vi "HFRR ADV v04.vi"() -> ()   [LabVIEW 2025] (continued)
            n1293 = Compound Arithmetic op=OR(w1606, w1605) -> (w1604:bool)
            n1294 = Not A Number/Path/Refnum?(number/path/refnum=w1590) -> (NaN/Path/Refnum?=w1601:bool)
            n1295 = case shown="True" w1604 {
              frame False {
              }
              frame True {
                n1296 = local write "TEMP"(0.0 ("TEMP")) -> ()
                n1297 = local write "FF 2"(0.0 ("FF 2")) -> ()
                n1298 = local write "reinit"(TRUE ("reinit")) -> ()
              }
            }
            n1299 = Select(t=0.0, s=w1601, f=w1590) -> (s? t:f=w1589:dbl)
            "COF 2" <- w1589
            n1300 = local write "COF 3"(w1589) -> ()
          }
        }
      }
    }
    n1301 = Wait (ms)(milliseconds to wait=u32 50) -> ()  [unwired: 1 out]
    n1302 = local read "Quit"() -> (w1529:bool)
    "Rate" <- 2500.0 ("No of Samples")
  }
  n1303 = while {
    tunnel: w57 -> [_]
    tunnel: [w1641] -> _
    tunnel: [w1617] -> w56
    i -> [w1641]
    stop <- w1617 stop-if-true
    # "C:\\LAB-IQ-NXT\\Scar View.exe"
    n1304 = local read "OK Button 16"() -> (w1630:bool)
    n1305 = local read "Main Tab"() -> (w1623:T2)
    n1306 = local read "service 3"() -> (w1624:bool)
    n1307 = local read "OPEN 6"() -> (w1626:bool)
    n1308 = local read "EDIT 2"() -> (w1628:bool)
    n1309 = flat-sequence {
      frame #0 {
        n1310 = local read "SAVE 2"() -> (w2243:bool)
        n1311 = stacked-sequence {
          frame #0 {
            n1312 = local read "EDIT"() -> (w2297:bool)
            n1313 = case shown="True" w2297 {
              tunnel: [u8 2 ("Disabled") u8 0 ("Disabled")] -> _
              frame False {
                w2299 = FALSE
                n1314 = local write "Password"("") -> ()
                n1315 = property on="SrvM CP" class="Bool (strict)"("Visible"=w2299) -> ()  [unwired: 2 in, 2 out]
                n1316 = property on="message" class="Str"("Visible"=w2299) -> ()  [unwired: 2 in, 2 out]
                n1317 = local write "x = y?"(w2299) -> ()
                n1318 = property on="Password" class="Str"("Visible"=w2299) -> ()  [unwired: 2 in, 2 out]
                n1319 = property on="ENTER THE NEW PASSWORD" class="Str"("Visible"=w2299) -> ()  [unwired: 2 in, 2 out]
                n1320 = property on="ENTER CURRENT PASSWORD" class="Str"("Visible"=w2299) -> ()  [unwired: 2 in, 2 out]
                n1321 = local write "SrvM CP"(w2299) -> ()
              }
              frame True {
                w2302 = TRUE
                n1322 = property on="SrvM CP" class="Bool (strict)"("Visible"=w2302) -> ()  [unwired: 2 in, 2 out]
                n1323 = property on="Password" class="Str"("Visible"=w2302) -> ()  [unwired: 2 in, 2 out]
              }
            }
            "dipl pwd" <- "@143$\n" ("dipl pwd")
          }
          frame #1 {
            # "Gain password"
            n1324 = String To Byte Array(string="ENTER CURRENT PASSWORD") -> (unsigned byte array=w2307:u8[])
            n1325 = Search 1D Array(1D array=w2307, element=u8 10) -> (index of element=w2310:i32)  [unwired: 1 in]
            n1326 = Index Array(array=w2307, index=w2310) -> (element=w2306:u8)
            n1327 = Equal?(x=w2306, y=10) -> (x = y?=w2304:bool)
            n1328 = case shown="True" w2304 {
              frame False {
                n1329 = property on="ENTER THE NEW PASSWORD" class="Str"("Visible"=FALSE) -> ()  [unwired: 2 in, 2 out]
              }
              frame True {
                # "password"
                # "change password logic"
                n1330 = local read "ENTER CURRENT PASSWORD"() -> (w2323:string)
                n1331 = local read "dipl pwd"() -> (w2317:string)
                n1332 = String To Byte Array(string=w2323) -> (unsigned byte array=w2325:u8[])
                n1333 = String To Byte Array(string=w2317) -> (unsigned byte array=w2318:u8[])
                n1334 = Array Size(array=w2325) -> (size(s)=w2322:i32)
                n1335 = Array Size(array=w2318) -> (size(s)=w2320:i32)
                n1336 = for {
                  N: w2322 -> [_]
                  tunnel: w2325 -> [w2349]
                  tunnel: [w2347] -> w2326 mode=indexing
                  tunnel: w2322 -> [w2341]
                  i -> [w2342]
                  n1337 = Decrement(x=w2341) -> (x-1=w2339:i32)
                  n1338 = Equal?(x=w2342, y=w2339) -> (x = y?=w2340:bool)
                  n1339 = Index Array(array=w2349, index=w2342) -> (element=w2343:u8)
                  n1340 = Number To Decimal String(number=w2343) -> (decimal integer string=w2348:string)  [unwired: 1 in]
                  n1341 = Select(t="", s=w2340, f="\r") -> (s? t:f=w2345:string)
                  n1342 = Concatenate Strings(w2348, w2345) -> (w2347:string)
                }
                n1343 = for {
                  N: w2320 -> [_]
                  tunnel: w2318 -> [w2337]
                  tunnel: [w2335] -> w2319 mode=indexing
                  tunnel: w2320 -> [w2332]
                  i -> [w2333]
                  n1344 = Decrement(x=w2332) -> (x-1=w2331:i32)
                  n1345 = Equal?(x=w2333, y=w2331) -> (x = y?=w2330:bool)
                  n1346 = Index Array(array=w2337, index=w2333) -> (element=w2336:u8)
                  n1347 = Number To Decimal String(number=w2336) -> (decimal integer string=w2334:string)  [unwired: 1 in]
                  n1348 = Select(t="", s=w2330, f="\r") -> (s? t:f=w2327:string)
                  n1349 = Concatenate Strings(w2334, w2327) -> (w2335:string)
                }
                n1350 = local read "string"() -> (w2324:string)
                n1351 = Concatenate Strings(w2319) -> (w2313:string)
                n1352 = Concatenate Strings(w2324) -> (w2321:string)
                n1353 = Concatenate Strings(w2326) -> (w2314:string)
                n1354 = Equal?(x=w2314, y=w2321) -> (x = y?=w2316:bool)
                n1355 = Equal?(x=w2314, y=w2313) -> (x = y?=w2312:bool)
                n1356 = Or(x=w2316, y=w2312) -> (x .or. y?=w2315:bool)
                n1357 = case shown="True" w2315 {
                  frame False {
                  }
                  frame True {
                    n1358 = property on="ENTER THE NEW PASSWORD" class="Str"("Visible"=TRUE) -> ()  [unwired: 2 in, 2 out]
                  }
                }
              }
            }
          }
          frame #2 {
            n1359 = String To Byte Array(string="ENTER THE NEW PASSWORD") -> (unsigned byte array=w2352:u8[])
            n1360 = Search 1D Array(1D array=w2352, element=u8 10) -> (index of element=w2356:i32)  [unwired: 1 in]
            n1361 = Index Array(array=w2352, index=w2356) -> (element=w2354:u8)
            n1362 = Equal?(x=w2354, y=10) -> (x = y?=w2351:bool)
            n1363 = case shown="False" w2351 {
              frame False {
              }
              frame True {
                n1364 = local write "EDIT"(FALSE) -> ()
                n1365 = local write "SrvM CP"(FALSE) -> ()
                n1366 = local read "ENTER THE NEW PASSWORD"() -> (w2359:string)
                n1367 = String To Byte Array(string=w2359) -> (unsigned byte array=w2364:u8[])
                n1368 = Array Size(array=w2364) -> (size(s)=w2361:i32)
                n1369 = for {
                  N: w2361 -> [_]
                  tunnel: w2364 -> [w2377]
                  tunnel: [w2374] -> w2366 mode=indexing
                  tunnel: w2361 -> [w2369]
                  i -> [w2367]
                  n1370 = Decrement(x=w2369) -> (x-1=w2370:i32)
                  n1371 = Equal?(x=w2367, y=w2370) -> (x = y?=w2371:bool)
                  n1372 = Index Array(array=w2377, index=w2367) -> (element=w2376:u8)
                  n1373 = Number To Decimal String(number=w2376) -> (decimal integer string=w2375:string)  [unwired: 1 in]
                  n1374 = Select(t="", s=w2371, f="\r") -> (s? t:f=w2368:string)
                  n1375 = Concatenate Strings(w2375, w2368) -> (w2374:string)
                }
                n1376 = local read "file path"() -> (w2358:path)
                n1377 = Concatenate Strings(w2366) -> (w2360:string)
                n1378 = Delete(path (use dialog)=w2358) -> (deleted path=w2362:path)  [unwired: 4 in, 2 out]
                n1379 = call <vilib>:"Write Characters To File.vi"("append to file? (new file:F)"=FALSE, "character string"=w2360, "file path (dialog if empty)"=w2362) -> ()  [unwired: 2 in, 1 out]
              }
            }
          }
          frame #3 {
            n1380 = case shown="True" "SrvM CP" {
              frame False {
                w2380 = ""
                n1381 = local write "ENTER CURRENT PASSWORD"(w2380) -> ()
                n1382 = local write "ENTER THE NEW PASSWORD"(w2380) -> ()
                n1383 = property on="ENTER CURRENT PASSWORD" class="Str"("Visible"=FALSE) -> ()  [unwired: 2 in, 2 out]
              }
              frame True {
                n1384 = property on="ENTER THE NEW PASSWORD" class="Str"() -> ("Visible"=w2381:bool)  [unwired: 2 in, 2 out]
                n1385 = Not(x=w2381) -> (.not. x?=w2382:bool)
                n1386 = property on="ENTER CURRENT PASSWORD" class="Str"("Visible"=w2382) -> ()  [unwired: 2 in, 2 out]
              }
            }
          }
          frame #4 {
            n1387 = String To Byte Array(string="Password") -> (unsigned byte array=w2389:u8[])
            n1388 = Search 1D Array(1D array=w2389, element=u8 10) -> (index of element=w2387:i32)  [unwired: 1 in]
            n1389 = Index Array(array=w2389, index=w2387) -> (element=w2388:u8)
            n1390 = Equal?(x=w2388, y=10) -> (x = y?=w2384:bool)
            n1391 = case shown="True" w2384 {
              frame False {
              }
              frame True {
                # "password"
                # "password"
                n1392 = local read "Password"() -> (w2402:string)
                n1393 = String To Byte Array(string=w2402) -> (unsigned byte array=w2405:u8[])
                n1394 = String To Byte Array(string="@143$\n") -> (unsigned byte array=w2391:u8[])
                n1395 = Array Size(array=w2405) -> (size(s)=w2400:i32)
                n1396 = Array Size(array=w2391) -> (size(s)=w2396:i32)
                n1397 = for {
                  N: w2400 -> [_]
                  tunnel: w2405 -> [w2439]
                  tunnel: [w2437] -> w2406 mode=indexing
                  tunnel: w2400 -> [w2434]
                  i -> [w2435]
                  n1398 = Decrement(x=w2434) -> (x-1=w2433:i32)
                  n1399 = Index Array(array=w2439, index=w2435) -> (element=w2438:u8)
                  n1400 = Equal?(x=w2435, y=w2433) -> (x = y?=w2432:bool)
                  n1401 = Number To Decimal String(number=w2438) -> (decimal integer string=w2436:string)  [unwired: 1 in]
                  n1402 = Select(t="", s=w2432, f="\r") -> (s? t:f=w2429:string)
                  n1403 = Concatenate Strings(w2436, w2429) -> (w2437:string)
                }
                n1404 = for {
                  N: w2396 -> [_]
                  tunnel: w2391 -> [w2450]
                  tunnel: [w2448] -> w2394 mode=indexing
                  tunnel: w2396 -> [w2445]
                  i -> [w2446]
                  n1405 = Decrement(x=w2445) -> (x-1=w2444:i32)
                  n1406 = Index Array(array=w2450, index=w2446) -> (element=w2449:u8)
                  n1407 = Equal?(x=w2446, y=w2444) -> (x = y?=w2443:bool)
                  n1408 = Number To Decimal String(number=w2449) -> (decimal integer string=w2447:string)  [unwired: 1 in]
                  n1409 = Select(t="", s=w2443, f="\r") -> (s? t:f=w2440:string)
                  n1410 = Concatenate Strings(w2447, w2440) -> (w2448:string)
                }
                n1411 = local read "file path"() -> (w2390:path)
                n1412 = call <vilib>:"Read Characters From File.vi"("file path (dialog if empty)"=w2390) -> ("character string"=w2404:string)  [unwired: 5 in, 3 out]
                "string" <- w2404
                n1413 = flat-sequence {
                  tunnel: [w2407] -> w2401
                  frame #0 {
                    w2407 = ""
                    n1414 = local write "Password"(w2407) -> ()
                  }
                }
                n1415 = Concatenate Strings(w2394) -> (w2395:string)
                n1416 = Concatenate Strings(w2404) -> (w2403:string)
                n1417 = Concatenate Strings(w2406) -> (w2398:string)
                n1418 = Equal?(x=w2398, y=w2403) -> (x = y?=w2393:bool)
                n1419 = Equal?(x=w2398, y=w2395) -> (x = y?=w2399:bool)
                n1420 = Or(x=w2393, y=w2399) -> (x .or. y?=w2392:bool)
                "x = y?" <- w2392
                n1421 = case shown="True" w2392 {
                  selector: w2392 -> [w2409 _]
                  tunnel: w2401 -> [_ _]
                  frame False {
                    n1422 = And(x=w2409, y=TRUE ("Visible")) -> (x .and. y?=w2410:bool)
                    n1423 = property on="message" class="Str"("Visible"=w2410) -> ()  [unwired: 2 in, 2 out]
                  }
                  frame True {
                    n1424 = control-ref of="This VI"() -> (w2421:refnum<vi>)
                    n1425 = property class="VI"(reference=w2421) -> (reference out=w2412:refnum<vi>, error out=w2416:errorcluster, "Panel"=w2420:refnum<vi>)  [unwired: 1 in]
                    n1426 = property on="message" class="Str"("Visible"=FALSE) -> ()  [unwired: 2 in, 2 out]
                    n1427 = property class="Pnl"(reference=w2420, error in=w2416) -> (reference out=w2414:refnum<vi>, error out=w2417:errorcluster, "Panes[]"=w2419:refnum<vi>[])
                    n1428 = for {
                      tunnel: w2419 -> [w2428] mode=indexing
                      tunnel: T15."Always On" ("Horizontal Scrollbar Visibility") -> [w2427]
                      tunnel: w2417 -> [w2424]
                      tunnel: [w2423] -> w2415
                      n1429 = property class="Pane"(reference=w2428, error in=w2424, "HorizScrollbarVisibility"=w2427) -> (reference out=w2425:refnum<vi>, error out=w2426:errorcluster)
                      n1430 = Close Reference(reference=w2425, error in (no error)=w2426) -> (error out=w2423:errorcluster)
                    }
                    n1431 = Close Reference(reference=w2414, error in (no error)=w2415) -> (error out=w2413:errorcluster)
                    n1432 = Close Reference(reference=w2412, error in (no error)=w2413) -> (error out=→"error out 6":errorcluster)
                  }
                }
              }
            }
          }
        }
        n1433 = local read "x = y?"() -> (w2249:bool)
        n1434 = local read "HUMIDITY: 2"() -> (w2251:dbl)
        n1435 = local read "HUMIDITY:"() -> (w2250:dbl)
        n1436 = property on="Port 2 Error" class="Clust (strict)"("Visible"="EDIT") -> ()  [unwired: 2 in, 2 out]
        n1437 = property on="Port 1 Error" class="Clust (strict)"("Visible"="EDIT") -> ()  [unwired: 2 in, 2 out]
        n1438 = case shown="True" "SrvM CP 2" {
          frame False {
          }
          frame True {
            n1439 = local write "SrvM CP 2"(FALSE ("SrvM CP 2")) -> ()
            n1440 = local read "HUMIDITY: 2"() -> (w2290:dbl)
            n1441 = local read "TEMP INTERCEPT: 2"() -> (w2289:dbl)
            n1442 = local read "DISPLACEMENT : 4"() -> (w2293:dbl)
            n1443 = local read "TEMPERATURE : 2"() -> (w2292:dbl)
            n1444 = local read "STROKE GAIN : 2"() -> (w2294:dbl)
            n1445 = local read "FRIC. FORCE : 2"() -> (w2295:dbl)
            n1446 = local read "AIR TEMP INTERCEPT: 2"() -> (w2288:dbl)
            n1447 = local read "AIR TEMPERATURE : 2"() -> (w2291:dbl)
            n1448 = local write "HUMIDITY:"(w2290) -> ()
            n1449 = local write "AIR TEMP INTERCEPT:"(w2289) -> ()
            n1450 = local write "TEMPERATURE :"(w2292) -> ()
            n1451 = local write "FRIC. FORCE :"(w2295) -> ()
            n1452 = local write "STROKE GAIN :"(w2294) -> ()
            n1453 = local write "DISPLACEMENT :"(w2293) -> ()
            n1454 = local write "AIR TEMPERATURE :"(w2291) -> ()
            n1455 = local write "TEMP INTERCEPT:"(w2288) -> ()
          }
        }
        n1456 = Or(x="SAVE", y=w2243) -> (x .or. y?=w2244:bool)
        n1457 = And(x="EDIT", y=w2249) -> (x .and. y?=w2247:bool)
        n1458 = local read "DISPLACEMENT : 4"() -> (w2260:dbl)
        n1459 = local read "TEMPERATURE : 2"() -> (w2258:dbl)
        n1460 = local read "STROKE GAIN : 2"() -> (w2264:dbl)
        n1461 = local read "DISPLACEMENT :"() -> (w2259:dbl)
        n1462 = local read "FRIC. FORCE : 2"() -> (w2267:dbl)
        n1463 = local read "TEMPERATURE :"() -> (w2256:dbl)
        n1464 = local read "STROKE GAIN :"() -> (w2263:dbl)
        n1465 = local read "FRIC. FORCE :"() -> (w2266:dbl)
        n1466 = case shown="True" w2247 {
          tunnel: [u8 2 ("Disabled") u8 0 ("Disabled")] -> w2246
          tunnel: [w2611 TRUE ("Visible")] -> w2245
          frame False {
            w2611 = FALSE ("Visible")
            n1467 = local write "EDIT 2"(w2611) -> ()
          }
          frame True {
          }
        }
        n1468 = case shown="True" w2244 {
          frame False {
          }
          frame True {
            n1469 = stacked-sequence {
              seq-local: [w2459 _ _] -> [_ w2606 _]
              frame #0 {
                (unwired) i16 5 ("precision (6)")
                # "[CH1]    - FF\n[CH2]   - TEMPERATURE\n[CH3]    - Humidity\n[CH4]    - AIR TEMP\n[CH5]\\- Visa Uno\n[CH6] \\- Visa Due\n[CH7]  \\- file path\n[CH8]   - Displacement Gain\n[CHA]   - Stroke Gain\n[CHB]   - Stroke PID Gain\n[CHC]   -Language Selection\n[CHD]   -Power +\n[CHE]   -Power_\n[CHF]   -Heater\n[CHG]   -Humidity Wet\n[CHH]   -Humidity Dry\n[CHI]   -Integral Time"
                n1470 = local read "Language Selection"() -> (w2507:enum16{"English", "Russian"})
                n1471 = local read "CH-HUMIDITY WET"() -> (w2465:u16)
                n1472 = local read "CH-HUMIDITY DRY"() -> (w2462:u16)
                n1473 = local read "STROKE GAIN :"() -> (w2451:dbl)
                n1474 = local read "CH-POWER +"() -> (w2474:u16)
                n1475 = local read "CH-POWER -"() -> (w2471:u16)
                n1476 = local read "CH-HEATER"() -> (w2468:u16)
                n1477 = local read "AIR TEMPERATURE :"() -> (w2454:dbl)
                n1478 = local read "DISPLACEMENT :"() -> (w2452:dbl)
                n1479 = local read "TEMPERATURE :"() -> (w2455:dbl)
                n1480 = local read "FRIC. FORCE :"() -> (w2456:dbl)
                n1481 = local read "HUMIDITY:"() -> (w2453:dbl)
                n1482 = Path To String(path="File Path") -> (string=w2523:string)
                n1483 = Number To Fractional String(number=w2451, width (-)=i16 10 ("precision (6)"), precision (6)=i16 5) -> (F-format string=w2514:string)  [unwired: 1 in]
                n1484 = Number To Fractional String(number=w2507, width (-)=i16 10 ("precision (6)"), precision (6)=i16 5) -> (F-format string=w2503:string)  [unwired: 1 in]
                n1485 = Number To Fractional String(number=w2474, width (-)=i16 10 ("precision (6)"), precision (6)=i16 5) -> (F-format string=w2497:string)  [unwired: 1 in]
                n1486 = Number To Fractional String(number=w2471, width (-)=i16 10 ("precision (6)"), precision (6)=i16 5) -> (F-format string=w2494:string)  [unwired: 1 in]
                n1487 = Number To Fractional String(number=w2468, width (-)=i16 10 ("precision (6)"), precision (6)=i16 5) -> (F-format string=w2489:string)  [unwired: 1 in]
                n1488 = Number To Fractional String(number=w2465, width (-)=i16 10 ("precision (6)"), precision (6)=i16 5) -> (F-format string=w2486:string)  [unwired: 1 in]
                n1489 = Number To Fractional String(number=w2462, width (-)=i16 10 ("precision (6)"), precision (6)=i16 5) -> (F-format string=w2481:string)  [unwired: 1 in]
                n1490 = local read "Com Port 1"() -> (w2458:refnum<visa-resource-name>)
                n1491 = local read "Com Port 2"() -> (w2457:refnum<visa-resource-name>)
                n1492 = Concatenate Strings(w2523, "\\" ("string")) -> (w2522:string)
                n1493 = Number To Fractional String(number=w2456, width (-)=i16 10 ("precision (6)"), precision (6)=i16 5) -> (F-format string=w2555:string)  [unwired: 1 in]
                n1494 = Number To Fractional String(number=w2455, width (-)=i16 10 ("precision (6)"), precision (6)=i16 5) -> (F-format string=w2554:string)  [unwired: 1 in]
                n1495 = Number To Fractional String(number=w2453, width (-)=i16 10 ("precision (6)"), precision (6)=i16 5) -> (F-format string=w2548:string)  [unwired: 1 in]
                n1496 = Number To Fractional String(number=w2454, width (-)=i16 10 ("precision (6)"), precision (6)=i16 5) -> (F-format string=w2542:string)  [unwired: 1 in]
                n1497 = Number To Fractional String(number=w2452, width (-)=i16 10 ("precision (6)"), precision (6)=i16 5) -> (F-format string=w2515:string)  [unwired: 1 in]
                n1498 = Concatenate Strings("[CHA]" ("string"), w2514, "- Stroke Gain" ("string"), "\r") -> (w2508:string)
                n1499 = Concatenate Strings("[CHC]" ("string"), w2503, "-Language Selection" ("string"), "\r") -> (w2500:string)
                n1500 = Concatenate Strings("[CHD]" ("string"), w2497, "-Power +" ("string"), "\r") -> (w2479:string)
                n1501 = Concatenate Strings("[CHG]" ("string"), w2486, "-Humidity Wet" ("string"), "\r") -> (w2476:string)
                n1502 = Concatenate Strings("[CHH]" ("string"), w2481, "-Humidity Dry" ("string"), "\r") -> (w2475:string)
                n1503 = Concatenate Strings("[CH1]" ("string"), w2555, " - FF" ("string"), "\r") -> (w2553:string)
                n1504 = Concatenate Strings("[CH2]" ("string"), w2554, " - TEMPERATURE" ("string"), "\r") -> (w2552:string)
                n1505 = Concatenate Strings("[CH3]" ("string"), w2548, " - Humidity" ("string"), "\r") -> (w2545:string)
                n1506 = Concatenate Strings("[CH4]" ("string"), w2542, " - AIR TEMP" ("string"), "\r") -> (w2538:string)
                n1507 = Concatenate Strings("[CH5]" ("string"), w2458, "- Visa Uno" ("string"), "\r") -> (w2531:string)
                n1508 = Concatenate Strings("[CH6]" ("string"), w2457, "- Visa Due" ("string"), "\r") -> (w2526:string)
                n1509 = Concatenate Strings("[CH7]" ("string"), w2522, "- file path" ("string"), "\r") -> (w2525:string)
                n1510 = Concatenate Strings("[CH8]" ("string"), w2515, "- Displacement Gain" ("string"), "\r") -> (w2518:string)
                n1511 = Concatenate Strings("[CHE]" ("string"), w2494, "-Power_" ("string"), "\r") -> (w2478:string)
                n1512 = Concatenate Strings("[CHF]" ("string"), w2489, "-Heater" ("string"), "\r") -> (w2477:string)
                n1513 = Concatenate Strings(w2553, w2552, w2545, w2538, w2531, w2526, w2525, w2518, w2508, w2500, w2479, w2478, w2477, w2476, w2475) -> (w2459:string)
                "gain" <- w2459
              }
              frame #1 {
                n1514 = local read "Camera Port :"() -> (w2567:string)
                n1515 = local read "C3 :"() -> (w2575:refnum<visa-resource-name>)
                n1516 = local read "TEMP INTERCEPT:"() -> (w2576:dbl)
                n1517 = local read "AIR TEMP INTERCEPT:"() -> (w2577:dbl)
                n1518 = Concatenate Strings("[CH8]" ("string"), w2567, "- Visa Camera" ("string"), "\r") -> (w2566:string)
                n1519 = Concatenate Strings("[CH7]" ("string"), w2575, "- Visa Humidity" ("string"), "\r") -> (w2571:string)
                n1520 = Number To Fractional String(number=w2576, width (-)=i16 10 ("precision (6)"), precision (6)=i16 5) -> (F-format string=w2594:string)  [unwired: 1 in]
                n1521 = local read "Com Port 3"() -> (w2578:refnum<visa-resource-name>)
                n1522 = Number To Fractional String(number=w2577, width (-)=i16 10 ("precision (6)"), precision (6)=i16 5) -> (F-format string=w2601:string)  [unwired: 1 in]
                n1523 = Concatenate Strings("[CHK]" ("string"), w2594, "-TEMP INTERCEPT" ("string"), "\r") -> (w2590:string)
                n1524 = Concatenate Strings("[SNO]" ("string"), "S.NO", "-" ("string"), "\r") -> (w2586:string)
                n1525 = Concatenate Strings("[CHJ]" ("string"), w2601, "-AIR TEMP INTERCEPT" ("string"), "\r") -> (w2591:string)
                n1526 = Concatenate Strings("[CHL]" ("string"), w2578, "- Visa humid" ("string"), "\r") -> (w2581:string)
                n1527 = String To Path(string="C:\\LAB-IQ\\calibrate WO 2465.dcf") -> (path=w2579:path)
                n1528 = Concatenate Strings(w2606, w2591, w2590, w2586, w2581, w2571, w2566) -> (w2605:string)
                n1529 = call <vilib>:"Write Characters To File.vi"("append to file? (new file:F)"=FALSE, "character string"=w2605, "file path (dialog if empty)"=w2579) -> ()  [unwired: 2 in, 1 out]
              }
              frame #2 {
                n1530 = local write "Lan flag"(0.0 ("Lan flag")) -> ()
                n1531 = local write "conststatus"(0.0 ("rpm value : 2")) -> ()
                n1532 = local write "SAVE"(FALSE ("OK Button 14")) -> ()
                n1533 = local write "SAVE 2"(FALSE ("SAVE 2")) -> ()
              }
            }
          }
        }
        n1534 = Subtract(x=w2251, y=w2250) -> (x-y=w2252:dbl)
        n1535 = local read "AIR TEMPERATURE : 2"() -> (w2255:dbl)
        n1536 = local read "AIR TEMPERATURE :"() -> (w2254:dbl)
        n1537 = Divide(x=w2252, y=w2250) -> (x/y=w2274:dbl)
        n1538 = Subtract(x=w2267, y=w2266) -> (x-y=w2265:dbl)
        n1539 = Subtract(x=w2258, y=w2256) -> (x-y=w2257:dbl)
        n1540 = Subtract(x=w2264, y=w2263) -> (x-y=w2262:dbl)
        n1541 = Subtract(x=w2260, y=w2259) -> (x-y=w2261:dbl)
        n1542 = Subtract(x=w2255, y=w2254) -> (x-y=w2253:dbl)
        n1543 = Divide(x=w2265, y=w2266) -> (x/y=w2285:dbl)
        n1544 = Divide(x=w2257, y=w2256) -> (x/y=w2278:dbl)
        n1545 = Divide(x=w2262, y=w2263) -> (x/y=w2282:dbl)
        n1546 = Divide(x=w2261, y=w2259) -> (x/y=w2281:dbl)
        n1547 = Multiply(x=w2274, y=100.0) -> (x*y=→"HUMIDITY  Calibration Error":dbl)
        n1548 = Divide(x=w2253, y=w2254) -> (x/y=w2277:dbl)
        n1549 = Multiply(x=w2285, y=100.0) -> (x*y=→"FRIC. FORCE Calibration Error":dbl)
        n1550 = Multiply(x=w2278, y=100.0) -> (x*y=→"TEMPERATURE  Calibration Error":dbl)
        n1551 = Multiply(x=w2282, y=100.0) -> (x*y=→"STROKE Calibration Error":dbl)
        n1552 = Multiply(x=w2281, y=100.0) -> (x*y=→"DISPLACEMENT  Calibration Error":dbl)
        n1553 = property on="EDIT 2" class="Bool (strict)"("Visible"=w2245) -> ()  [unwired: 2 in, 2 out]
        n1554 = property on="SAVE" class="Bool (strict)"("Visible"=w2245) -> ()  [unwired: 2 in, 2 out]
        n1555 = property on="SrvM CP" class="Bool (strict)"("Disabled"=w2246) -> ()  [unwired: 2 in, 2 out]
        n1556 = property on="visa due" class="CmbBox"("Disabled"=w2246) -> ()  [unwired: 2 in, 2 out]
        n1557 = property on="File Path" class="Path"("Disabled"=w2246) -> ()  [unwired: 2 in, 2 out]
        n1558 = Multiply(x=w2277, y=100.0) -> (x*y=→"AIR TEMPERATURE  Calibration Error":dbl)
        n1559 = property on="Language Selection" class="Enum (strict)"("Visible"=w2245) -> ()  [unwired: 2 in, 2 out]
        n1560 = property on="Tab Control 7" class="TabCtl (strict)"("Disabled"=w2246) -> ()  [unwired: 2 in, 2 out]
        n1561 = property on="AIR TEMP INTERCEPT:" class="DigNum (strict)"("Disabled"=w2246) -> ()  [unwired: 2 in, 2 out]
        n1562 = property on="CH-POWER -" class="DigNum (strict)"("Disabled"=w2246) -> ()  [unwired: 2 in, 2 out]
        n1563 = property on="CH-POWER +" class="DigNum (strict)"("Disabled"=w2246) -> ()  [unwired: 2 in, 2 out]
        n1564 = property on="AIR TEMPERATURE :" class="DigNum (strict)"("Disabled"=w2246) -> ()  [unwired: 2 in, 2 out]
        n1565 = property on="STROKE GAIN :" class="DigNum (strict)"("Disabled"=w2246) -> ()  [unwired: 2 in, 2 out]
        n1566 = property on="SPEED OUT:" class="DigNum (strict)"("Disabled"=w2246) -> ()  [unwired: 2 in, 2 out]
        n1567 = property on="CH-HUMIDITY DRY" class="DigNum (strict)"("Disabled"=w2246) -> ()  [unwired: 2 in, 2 out]
        n1568 = property on="HUMIDITY:" class="DigNum (strict)"("Disabled"=w2246) -> ()  [unwired: 2 in, 2 out]
        n1569 = property on="CH-HUMIDITY WET" class="DigNum (strict)"("Disabled"=w2246) -> ()  [unwired: 2 in, 2 out]
        n1570 = property on="TEMPERATURE :" class="DigNum (strict)"("Disabled"=w2246) -> ()  [unwired: 2 in, 2 out]
        n1571 = property on="DISPLACEMENT :" class="DigNum (strict)"("Disabled"=w2246) -> ()  [unwired: 2 in, 2 out]
        n1572 = property on="CH-HEATER" class="DigNum (strict)"("Disabled"=w2246) -> ()  [unwired: 2 in, 2 out]
        n1573 = property on="TEMP INTERCEPT:" class="DigNum (strict)"("Disabled"=w2246) -> ()  [unwired: 2 in, 2 out]
        n1574 = property on="FRIC. FORCE :" class="DigNum (strict)"("Disabled"=w2246) -> ()  [unwired: 2 in, 2 out]
      }
    }
    n1575 = local read "RUN"() -> (w1640:bool)
    n1576 = local read "RUN"() -> (w1638:bool)
    n1577 = disable-structure shown="Disabled" {
      disable-tunnel: [w1655 _] -> w1621
      disable-tunnel: [w1654 _] -> w1619
      frame Disabled {
        n1578 = local read "Temperature before test"() -> (w1648:dbl)
        n1579 = local read "Temperature after test"() -> (w1661:dbl)
        n1580 = case shown="True" "Save Results" {
          frame False {
          }
          frame True {
            w1677 = "\r"
            n1581 = local write "Save Results"(FALSE ("OK Button 5")) -> ()
            n1582 = local read "Temperature before test"() -> (w1715:dbl)
            n1583 = local read "Temperature after test"() -> (w1717:dbl)
            n1584 = local read "Humidity before test"() -> (w1714:dbl)
            n1585 = local read "Humidity after test"() -> (w1716:dbl)
            n1586 = local read "WS1.4"() -> (w1721:dbl)
            n1587 = local read "AVP"() -> (w1719:dbl)
            n1588 = Number To Fractional String(number=w1721, width (-)=i16 6, precision (6)=i16 1) -> (F-format string=w1681:string)  [unwired: 1 in]
            n1589 = local read "MWSD"() -> (w1718:dbl)
            n1590 = local read "String"() -> (w1710:string)
            n1591 = local read "FILE"() -> (w1713:string)
            n1592 = local read "HCF"() -> (w1720:dbl)
            n1593 = Number To Fractional String(number=w1714, width (-)=i16 6, precision (6)=i16 1) -> (F-format string=w1706:string)  [unwired: 1 in]
            n1594 = Number To Fractional String(number=w1715, width (-)=i16 6, precision (6)=i16 1) -> (F-format string=w1703:string)  [unwired: 1 in]
            n1595 = Number To Fractional String(number=w1716, width (-)=i16 6, precision (6)=i16 1) -> (F-format string=w1699:string)  [unwired: 1 in]
            n1596 = Number To Fractional String(number=w1717, width (-)=i16 6, precision (6)=i16 1) -> (F-format string=w1695:string)  [unwired: 1 in]
            n1597 = Number To Fractional String(number=w1719, width (-)=i16 6, precision (6)=i16 3) -> (F-format string=w1688:string)  [unwired: 1 in]
            n1598 = Concatenate Strings(w1710, w1713) -> (w1732:string)
            n1599 = Number To Fractional String(number=w1718, width (-)=i16 6, precision (6)=i16 1) -> (F-format string=w1692:string)  [unwired: 1 in]
            n1600 = Number To Fractional String(number=w1720, width (-)=i16 6, precision (6)=i16 2) -> (F-format string=w1686:string)  [unwired: 1 in]
            n1601 = Concatenate Strings("(" ("string"), w1681, ")Microns" ("string")) -> (w1680:string)
            n1602 = local read "REMARKS"() -> (w1712:string)
            "REMARKS 2" <- w1712
            n1603 = Concatenate Strings("(" ("string"), w1706, " ) % RH," ("string")) -> (w1707:string)
            n1604 = Concatenate Strings(w1686, ")" ("string")) -> (w1684:string)
            n1605 = Concatenate Strings("(" ("string"), w1703, ")  Deg C ," ("string")) -> (w1702:string)
            n1606 = Concatenate Strings("(" ("string"), w1699, " ) % RH," ("string")) -> (w1698:string)
            n1607 = Concatenate Strings("(" ("string"), w1695, ")  Deg C ," ("string")) -> (w1694:string)
            n1608 = Concatenate Strings("(" ("string"), w1692, ")  Microns," ("string")) -> (w1691:string)
            n1609 = Concatenate Strings("(" ("string"), w1688, ")  kPa," ("string")) -> (w1678:string)
            n1610 = Concatenate Strings(w1732, ".dwm" ("Substring")) -> (w1730:string)
            n1611 = String To Path(string=w1730) -> (path=w1729:path)
            n1612 = Concatenate Strings(w1712, w1677, " Humidity before test= " ("Substring"), w1707, w1677, " Temperature before test = " ("Substring"), w1702, w1677, " Humidity after test= " ("Substring"), w1698, w1677, "Temperature after test = " ("Substring"), w1694, w1677, "MSD = " ("Substring"), w1691, w1677, "  AVP = " ("Substring"), w1678, w1677, "  HCF                     =( " ("Substring"), w1684, w1677, " WS1.4                  = " ("Substring"), w1680, w1677) -> (w1676:string)
            "data" <- w1676
            n1613 = call <vilib>:"Write Characters To File.vi"("append to file? (new file:F)"=FALSE, "character string"=w1676, "file path (dialog if empty)"=w1729) -> ()  [unwired: 2 in, 1 out]
            n1614 = Match Pattern(string=w1676, regular expression="!") -> (after substring=→"export":string)  [unwired: 1 in, 3 out]
          }
        }
        n1615 = Add(x=231.864, y=w1648) -> (x+y=w1645:dbl)
        n1616 = Add(x=231.864, y=w1661) -> (x+y=w1658:dbl)
        n1617 = Divide(x=1705.984, y=w1645) -> (x/y=w1646:dbl)
        n1618 = Divide(x=1705.984, y=w1658) -> (x/y=w1659:dbl)
        n1619 = local read "Humidity before test"() -> (w1650:dbl)
        n1620 = local read "Humidity after test"() -> (w1663:dbl)
        n1621 = Subtract(x=8.017352 ("y"), y=w1646) -> (x-y=w1672:dbl)
        n1622 = Subtract(x=8.017352 ("y"), y=w1659) -> (x-y=w1666:dbl)
        n1623 = expression code="10**y"(w1672) -> (w1652:dbl)
        n1624 = expression code="10**y"(w1666) -> (w1665:dbl)
        n1625 = Multiply(x=w1650, y=w1652) -> (x*y=w1651:dbl)
        n1626 = Multiply(x=w1663, y=w1665) -> (x*y=w1664:dbl)
        n1627 = Divide(x=w1651, y=750.0) -> (x/y=w1667:dbl)
        n1628 = Divide(x=w1664, y=750.0) -> (x/y=w1668:dbl)
        n1629 = Add(x=w1667, y=w1668) -> (x+y=w1669:dbl)
        n1630 = Divide(x=w1669, y=2.0) -> (x/y=w1671:dbl)
        n1631 = local write "AVP"(w1671) -> ()
        n1632 = Subtract(x=1.4, y=w1671) -> (x-y=w1654:dbl)
        n1633 = local read "HCF"() -> (w1655:dbl)
      }
      frame Enabled {
      }
    }
    n1634 = case shown="True" "EDIT 3" {
      frame False {
      }
      frame True {
        n1635 = local write "EDIT 3"(FALSE ("EDIT 3")) -> ()
        n1636 = local write "Main Tab"(T2."About" ("Main Tab")) -> ()
      }
    }
    n1637 = case shown="False" w1640 {
      frame False {
        n1638 = local read "stopT"() -> (w2618:bool)
        n1639 = case shown="True" w2618 {
          frame False {
          }
          frame True {
            n1640 = local write "stopT"(FALSE) -> ()
          }
        }
      }
      frame True {
        "stopT" <- TRUE
      }
    }
    n1641 = case shown="False" w1638 {
      frame False {
      }
      frame True {
      }
    }
    n1642 = case shown="True" w1628 {
      frame False {
        n1643 = property on="Password 2" class="Str"("Visible"=FALSE) -> ()  [unwired: 2 in, 2 out]
        n1644 = local write "Password 2"("" ("Password")) -> ()
      }
      frame True {
        n1645 = property on="Password 2" class="Str"("Visible"=TRUE) -> ()  [unwired: 2 in, 2 out]
        n1646 = Equal?(x="Password 2", y="HFRR1234") -> (x = y?=w1760:bool)
        n1647 = case shown="True" w1760 {
          tunnel: "Password 2" -> [w1763 _]
          frame False {
            n1648 = String Length(string=w1763) -> (length=w1764:i32)
            n1649 = Greater Than 0?(x=w1764) -> (x > 0?=w1762:bool)
            n1650 = case shown="False" w1762 {
              frame False {
                n1651 = property on="Password 2" class="Str"("Caption.Text"="Password (Advance Setting)") -> ()  [unwired: 2 in, 2 out]
              }
              frame True {
                n1652 = property on="Password 2" class="Str"("Caption.Text"="Incorrect Password!") -> ()  [unwired: 2 in, 2 out]
              }
            }
          }
          frame True {
            n1653 = local write "EDIT 2"(FALSE ("EDIT 2")) -> ()
            n1654 = local write "Password 2"("" ("Password")) -> ()
            n1655 = local write "Main Tab"(T2."Advance" ("Main Tab")) -> ()
            n1656 = local write "Main Dashboard Buttons"(T1."Advance" ("Main Dashboard Buttons")) -> ()
          }
        }
      }
    }
    n1657 = case shown="True" "Prog Uno" {
      frame False {
      }
      frame True {
        n1658 = stacked-sequence {
          frame #0 {
            n1659 = Delete(path (use dialog)=path "C:/LAB-IQ-NXT/UNOCOMPILE.bat" ("working directory")) -> ()  [unwired: 4 in, 3 out]
          }
          frame #1 {
            n1660 = local read "Com Port 1"() -> (w2225:refnum<visa-resource-name>)
            n1661 = Concatenate Strings("cmd.exe /c \"mode " ("command line"), w2225, ":1200,n,8,1\"\n" ("command line")) -> (w2230:string)
            n1662 = Concatenate Strings(w2230, "CD\\\nCD WinDucom\navrdude -C avrdude.conf -v -patmega328p -carduino -P" ("command line"), w2225, " -b115200 -D -Uflash:w:UNO_V20.hex:i\n" ("command line"), "\r") -> (w2232:string)
            "STR" <- w2232
            n1663 = call <vilib>:"Write Characters To File.vi"("append to file? (new file:F)"=FALSE, "character string"=w2232, "file path (dialog if empty)"=path "C:/LAB-IQ/UNOCOMPILE.bat" ("working directory")) -> ()  [unwired: 2 in, 1 out]
          }
          frame #2 {
            n1664 = disable-structure shown="Disabled" {
              frame Disabled {
                w2236 = "cmd.exe  /c \"C:\\LAB-IQ-NXT\\UNOCOMPILE.bat\"" ("string")
                n1665 = local write "Prog Uno"(FALSE ("run minimized? (F)")) -> ()
                n1666 = call <vilib>:"System Exec.vi"("expected output size  (4096)"=u32 65535, "run minimized? (F)"=FALSE, "wait until completion? (T)"=TRUE ("run minimized? (F)"), "working directory"=path "C:/LAB-IQ-NXT", "standard input"=w2236, "command line"=w2236) -> ("error out"=w2235:errorcluster, "standard output"=→"String 42":string)  [unwired: 2 in, 2 out]
                "error out 3" <- w2235
                n1667 = flat-sequence {
                  tunnel: w2235 -> [_]
                  frame #0 {
                  }
                }
              }
              frame Enabled {
              }
            }
          }
        }
      }
    }
    n1668 = case shown="\"CEC F-096-A-06\"" "TEST STANDARD" {
      tunnel: [2.0 ("Set Temp") 0.0 ("Set Temp") 2.0 ("Set Temp") 0.0 ("Set Temp")] -> w1629
      frame "ASTM D6079", Default {
        w2182 = 50.0 ("Hz")
        w2183 = 53.0 ("Set Rh")
        w2185 = 1.0 ("Set Strk")
        w2184 = 60.0 ("Set Temp")
        # "astm hide"
        n1669 = local write "NORMAL LOAD"(200.0 ("NORMAL LOAD")) -> ()
        n1670 = local write "Set Strk"(w2185) -> ()
        n1671 = local write "Set Hz"(w2182) -> ()
        n1672 = local write "Set Temp"(w2184) -> ()
        n1673 = local write "Set Rh"(w2183) -> ()
        n1674 = local write "test time"(75.0 ("test time")) -> ()
        n1675 = local write "Set Stroke:"(w2185) -> ()
        n1676 = local write "Set Humidity:"(w2183) -> ()
        n1677 = local write "Set Frequency:"(w2182) -> ()
        n1678 = local write "Set Temperature:"(w2184) -> ()
        "Test Standard" <- "ASTM D6079" ("Test Standard 2")
      }
      frame "ISO 12156" {
        n1679 = local write "Set Strk"(1.0 ("Set Strk")) -> ()
        n1680 = local write "NORMAL LOAD"(200.0 ("NORMAL LOAD")) -> ()
        n1681 = local write "Set Temp"(60.0 ("Set Temp")) -> ()
        n1682 = local write "test time"(75.0 ("test time")) -> ()
        n1683 = local write "Set Hz"(50.0 ("Hz")) -> ()
        n1684 = local write "Set Rh"(53.0 ("Set Rh")) -> ()
      }
      frame "CEC F-096-A-06" {
        n1685 = local write "Set Strk"(1.0 ("Set Strk")) -> ()
        n1686 = local write "NORMAL LOAD"(200.0 ("NORMAL LOAD")) -> ()
        n1687 = local write "Set Temp"(60.0 ("Set Temp")) -> ()
        n1688 = local write "test time"(75.0 ("test time")) -> ()
        n1689 = local write "Set Hz"(50.0 ("Hz")) -> ()
        n1690 = local write "Set Rh"(53.0 ("Set Rh")) -> ()
      }
      frame "Custom" {
      }
    }
    n1691 = case shown="True" "Prog Due" {
      frame False {
      }
      frame True {
        n1692 = stacked-sequence {
          frame #0 {
            n1693 = Delete(path (use dialog)=path "C:/LAB-IQ/DUECOMPILE.bat" ("working directory")) -> ()  [unwired: 4 in, 3 out]
          }
          frame #1 {
            n1694 = disable-structure shown="Disabled" {
              frame Disabled {
                n1695 = local read "visa due"() -> (w2207:string)
                n1696 = Concatenate Strings("cmd.exe /c \"mode " ("command line"), w2207, ":1200,n,8,1\"\n" ("command line")) -> (w2212:string)
                n1697 = Concatenate Strings(w2212, "CD\\\nCD WinDucom\nTIMEOUT 1\n bossac.exe -i -d --port=" ("command line"), w2207, " -U false -e -w -v -b DUE.bin -R\n" ("command line"), "\r") -> (w2214:string)
                "concatenated string 2" <- w2214
                n1698 = call <vilib>:"Write Characters To File.vi"("append to file? (new file:F)"=FALSE, "character string"=w2214, "file path (dialog if empty)"=path "C:/LAB-IQ-NXT/DUECOMPILE.bat" ("working directory")) -> ()  [unwired: 2 in, 1 out]
              }
              frame Enabled {
              }
            }
          }
          frame #2 {
            # "C:\\LAB-IQ-NXT\\DUECOMPILE.bat"
            n1699 = disable-structure shown="Disabled" {
              frame Disabled {
                w2219 = "cmd.exe  /c \"C:\\LAB-IQ-NXT\\DUECOMPILE.bat\"" ("string")
                n1700 = call <vilib>:"System Exec.vi"("expected output size  (4096)"=u32 65535, "run minimized? (F)"=FALSE, "wait until completion? (T)"=TRUE ("run minimized? (F)"), "working directory"=path "C:/LAB-IQ-NXT", "standard input"=w2219, "command line"=w2219) -> ("error out"=w2218:errorcluster, "standard output"=→"String 44":string)  [unwired: 2 in, 2 out]
                "error out 4" <- w2218
                n1701 = flat-sequence {
                  tunnel: w2218 -> [_]
                  frame #0 {
                  }
                }
              }
              frame Enabled {
              }
            }
            n1702 = local write "Prog Due"(FALSE ("Prog Due")) -> ()
          }
        }
      }
    }
    n1703 = Or(x=w1626, y=w1624) -> (x .or. y?=w1625:bool)
    n1704 = case shown="\"About\"" w1623 {
      tunnel: [T20."Acquire" ("Main Tab") T20."Compare Files" ("Main Tab") T20."About" ("Main Tab")] -> w1636
      frame "Acquire", Default {
      }
      frame "Compare Files" {
      }
      frame "About" {
      }
    }
    n1705 = Or(x=w1630, y="OPEN") -> (x .or. y?=w1631:bool)
    n1706 = case shown="True" w1631 {
      tunnel: w1630 -> [_ w1771]
      frame False {
      }
      frame True {
        n1707 = stacked-sequence {
          tunnel: w1771 -> [_ w1838 _ _]
          frame #0 {
            w1787 = "  " ("String 6")
            n1708 = local write "OPEN"(FALSE ("open")) -> ()
            n1709 = local read "string1 2"() -> (w1775:string)
            n1710 = local read "string1 3"() -> (w1774:string)
            n1711 = local read "string1 4"() -> (w1773:string)
            n1712 = property on="OPEN" class="Bool (strict)"("Visible"=FALSE) -> ()  [unwired: 2 in, 2 out]
            n1713 = local write "String 6"(w1787) -> ()
            n1714 = local write "String 7"(w1787) -> ()
            n1715 = local write "String 8"(w1787) -> ()
            n1716 = local write "String 12"(w1787) -> ()
            n1717 = local read "OK Button 16"() -> (w1772:bool)
            n1718 = String To Path(string=w1775) -> (path=w1783:path)
            n1719 = String To Path(string=w1774) -> (path=w1782:path)
            n1720 = String To Path(string=w1773) -> (path=w1781:path)
            n1721 = case shown="True" w1772 {
              tunnel: [w1788 w1789] -> w1776
              frame False {
                n1722 = local read "string1"() -> (w1788:string)
              }
              frame True {
                n1723 = local read "String Indicator 4"() -> (w1789:string)
              }
            }
            n1724 = Open/Create/Replace File "Open File"(file path (use dialog)=w1783) -> (refnum out=w1779:refnum<file>)  [unwired: 5 in, 2 out]
            n1725 = Open/Create/Replace File "Open File"(file path (use dialog)=w1782) -> (refnum out=w1778:refnum<file>)  [unwired: 5 in, 2 out]
            n1726 = Open/Create/Replace File "Open File"(file path (use dialog)=w1781) -> (refnum out=w1777:refnum<file>)  [unwired: 5 in, 2 out]
            n1727 = while {
              tunnel: w1779 -> [w1801]
              i -> [w1797]
              stop <- w1796 continue-if-true
              (unwired) TRUE ("line mode (F)")
              n1728 = Read from Text File "Read File"(file (use dialog)=w1801) -> (text=w1798:string)  [unwired: 3 in, 3 out]
              n1729 = local write "Numeric 11"(w1797) -> ()
              n1730 = String Length(string=w1798) -> (length=w1800:i32)
              n1731 = Greater?(x=w1800, y=1) -> (0:w1796:bool)
            }
            n1732 = while {
              tunnel: w1778 -> [w1807]
              i -> [w1803]
              stop <- w1802 continue-if-true
              (unwired) TRUE ("line mode (F)")
              n1733 = Read from Text File "Read File"(file (use dialog)=w1807) -> (text=w1804:string)  [unwired: 3 in, 3 out]
              n1734 = local write "Numeric 12"(w1803) -> ()
              n1735 = String Length(string=w1804) -> (length=w1806:i32)
              n1736 = Greater?(x=w1806, y=1) -> (0:w1802:bool)
            }
            n1737 = while {
              tunnel: w1777 -> [w1813]
              i -> [w1809]
              stop <- w1808 continue-if-true
              (unwired) TRUE ("line mode (F)")
              n1738 = Read from Text File "Read File"(file (use dialog)=w1813) -> (text=w1810:string)  [unwired: 3 in, 3 out]
              n1739 = local write "Numeric 13"(w1809) -> ()
              n1740 = String Length(string=w1810) -> (length=w1812:i32)
              n1741 = Greater?(x=w1812, y=1) -> (0:w1808:bool)
            }
            n1742 = String To Path(string=w1776) -> (path=w1784:path)
            n1743 = Open/Create/Replace File "Open File"(file path (use dialog)=w1784) -> (refnum out=w1780:refnum<file>)  [unwired: 5 in, 2 out]
            n1744 = while {
              tunnel: w1780 -> [w1795]
              i -> [w1791]
              stop <- w1790 continue-if-true
              (unwired) TRUE ("line mode (F)")
              n1745 = Read from Text File "Read File"(file (use dialog)=w1795) -> (text=w1792:string)  [unwired: 3 in, 3 out]
              n1746 = local write "Numeric 8"(w1791) -> ()
              n1747 = String Length(string=w1792) -> (length=w1794:i32)
              n1748 = Greater?(x=w1794, y=1) -> (0:w1790:bool)
            }
          }
          frame #1 {
            w1965 = FALSE ("ACTUAL   MERGE")
            # "Sample Temp"
            # "ECR"
            # "COF"
            # "Time\nCOF\nFF\nTemp"
            n1749 = case shown="True" w1838 {
              tunnel: [w1985 w1986] -> w1839
              frame False {
                n1750 = local read "string1"() -> (w1985:string)
              }
              frame True {
                n1751 = local read "String Indicator 4"() -> (w1986:string)
              }
            }
            n1752 = local read "string1 3"() -> (w1883:string)
            n1753 = String To Path(string=w1839) -> (path=w1970:path)
            n1754 = String To Path(string=w1883) -> (path=w1981:path)
            n1755 = local read "Numeric 12"() -> (w1967:i32)
            n1756 = local read "Numeric 8"() -> (w1969:i32)
            n1757 = local read "string1 2"() -> (w1884:string)
            n1758 = local read "string1 4"() -> (w1882:string)
            n1759 = Open/Create/Replace File "Open File"(file path (use dialog)=w1970) -> (refnum out=w1984:refnum<file>, error out=w1983:errorcluster)  [unwired: 5 in, 1 out]
            n1760 = Open/Create/Replace File "Open File"(file path (use dialog)=w1981) -> (refnum out=w1977:refnum<file>, error out=w1978:errorcluster)  [unwired: 5 in, 1 out]
            n1761 = for {
              N: w1969 -> [_]
              tunnel: w1984 -> [w2132]
              tunnel: w1983 -> [w2131]
              tunnel: [w2121] -> w1896 mode=indexing
              tunnel: [w2119] -> w1953 mode=indexing
              tunnel: [w2120] -> w1948 mode=indexing
              tunnel: w1965 -> [_]
              tunnel: [w2113] -> w1950 mode=indexing
              tunnel: [w2109] -> w1919 mode=indexing
              tunnel: [w2105] -> w1894 mode=indexing
              tunnel: [w2101] -> w1875 mode=indexing
              tunnel: [w2096] -> w1835 mode=indexing
              (unwired) TRUE ("line mode (F)")
              # "freq"
              # "Stroke"
              # "Time"
              # "CoF"
              # "Humidity"
              # "Temp"
              # "Air Temp"
              # "ECR"
              n1762 = Read from Text File "Read File"(file (use dialog)=w2132, error in=w2131) -> (text=w2097:string)  [unwired: 2 in, 3 out]
              n1763 = local write "String 6"(w2097) -> ()
              n1764 = String Subset(string=w2097, offset (0)=0, length (rest)=14 ("length (rest)")) -> (substring=w2125:string)
              n1765 = String Subset(string=w2097, offset (0)=35, length (rest)=9 ("length (rest)")) -> (substring=w2122:string)
              n1766 = String Subset(string=w2097, offset (0)=15, length (rest)=9 ("length (rest)")) -> (substring=w2128:string)
              n1767 = Fract/Exp String To Number(string=w2125) -> (number=w2121:dbl)  [unwired: 3 in, 1 out]
              n1768 = Fract/Exp String To Number(string=w2122) -> (number=w2120:dbl)  [unwired: 3 in, 1 out]
              n1769 = Fract/Exp String To Number(string=w2128) -> (number=w2119:dbl)  [unwired: 3 in, 1 out]
              n1770 = String Subset(string=w2097, offset (0)=85, length (rest)=9 ("length (rest)")) -> (substring=w2098:string)
              n1771 = String Subset(string=w2097, offset (0)=25, length (rest)=9 ("length (rest)")) -> (substring=w2104:string)
              n1772 = String Subset(string=w2097, offset (0)=55, length (rest)=9 ("length (rest)")) -> (substring=w2106:string)
              n1773 = String Subset(string=w2097, offset (0)=45, length (rest)=9 ("length (rest)")) -> (substring=w2112:string)
              n1774 = String Subset(string=w2097, offset (0)=65, length (rest)=9 ("length (rest)")) -> (substring=w2118:string)
              n1775 = Fract/Exp String To Number(string=w2104) -> (number=w2101:dbl)  [unwired: 3 in, 1 out]
              n1776 = Fract/Exp String To Number(string=w2098) -> (number=w2096:dbl)  [unwired: 3 in, 1 out]
              n1777 = Fract/Exp String To Number(string=w2106) -> (number=w2105:dbl)  [unwired: 3 in, 1 out]
              n1778 = Fract/Exp String To Number(string=w2112) -> (number=w2109:dbl)  [unwired: 3 in, 1 out]
              n1779 = Fract/Exp String To Number(string=w2118) -> (number=w2115:dbl)  [unwired: 3 in, 1 out]
              n1780 = Add(x=w2115, y=0.0) -> (x+y=w2113:dbl)
            }
            n1781 = for {
              N: w1967 -> [_]
              tunnel: w1978 -> [w2058]
              tunnel: w1977 -> [w2057]
              tunnel: [w2047] -> w1936 mode=indexing
              tunnel: [w2045] -> w1934 mode=indexing
              tunnel: [w2046] -> w1930 mode=indexing
              tunnel: w1965 -> [_]
              tunnel: [w2039] -> w1932 mode=indexing
              tunnel: [w2035] -> w1914 mode=indexing
              tunnel: [w2031] -> w1890 mode=indexing
              tunnel: [w2028] -> w1871 mode=indexing
              tunnel: [w2024] -> w1830 mode=indexing
              (unwired) 9 ("length (rest)")
              (unwired) 9 ("length (rest)")
              (unwired) TRUE ("line mode (F)")
              n1782 = Read from Text File "Read File"(file (use dialog)=w2057, error in=w2058) -> (text=w2025:string)  [unwired: 2 in, 3 out]
              n1783 = local write "String 8"(w2025) -> ()
              n1784 = String Subset(string=w2025, offset (0)=85) -> (substring=w2027:string)  [unwired: 1 in]
              n1785 = String Subset(string=w2025, offset (0)=35, length (rest)=9 ("length (rest)")) -> (substring=w2048:string)
              n1786 = String Subset(string=w2025, offset (0)=55, length (rest)=9 ("length (rest)")) -> (substring=w2033:string)
              n1787 = String Subset(string=w2025, offset (0)=25) -> (substring=w2029:string)  [unwired: 1 in]
              n1788 = String Subset(string=w2025, offset (0)=15, length (rest)=9 ("length (rest)")) -> (substring=w2054:string)
              n1789 = String Subset(string=w2025, offset (0)=0, length (rest)=14 ("length (rest)")) -> (substring=w2051:string)
              n1790 = String Subset(string=w2025, offset (0)=45, length (rest)=9 ("length (rest)")) -> (substring=w2038:string)
              n1791 = String Subset(string=w2025, offset (0)=65, length (rest)=9 ("length (rest)")) -> (substring=w2044:string)
              n1792 = Fract/Exp String To Number(string=w2027) -> (number=w2024:dbl)  [unwired: 3 in, 1 out]
              n1793 = Fract/Exp String To Number(string=w2048) -> (number=w2046:dbl)  [unwired: 3 in, 1 out]
              n1794 = Fract/Exp String To Number(string=w2033) -> (number=w2031:dbl)  [unwired: 3 in, 1 out]
              n1795 = Fract/Exp String To Number(string=w2029) -> (number=w2028:dbl)  [unwired: 3 in, 1 out]
              n1796 = Fract/Exp String To Number(string=w2054) -> (number=w2045:dbl)  [unwired: 3 in, 1 out]
              n1797 = Fract/Exp String To Number(string=w2051) -> (number=w2047:dbl)  [unwired: 3 in, 1 out]
              n1798 = Fract/Exp String To Number(string=w2038) -> (number=w2035:dbl)  [unwired: 3 in, 1 out]
              n1799 = Fract/Exp String To Number(string=w2044) -> (number=w2041:dbl)  [unwired: 3 in, 1 out]
              n1800 = Add(x=w2041, y=0.0) -> (x+y=w2039:dbl)
            }
            n1801 = String To Path(string=w1884) -> (path=w1982:path)
            n1802 = String To Path(string=w1882) -> (path=w1976:path)
            n1803 = local read "Numeric 11"() -> (w1966:i32)
            n1804 = local read "Numeric 13"() -> (w1968:i32)
            n1805 = Open/Create/Replace File "Open File"(file path (use dialog)=w1982) -> (refnum out=w1980:refnum<file>, error out=w1979:errorcluster)  [unwired: 5 in, 1 out]
            n1806 = Open/Create/Replace File "Open File"(file path (use dialog)=w1976) -> (refnum out=w1975:refnum<file>, error out=w1974:errorcluster)  [unwired: 5 in, 1 out]
            n1807 = for {
              N: w1966 -> [_]
              tunnel: w1980 -> [w2095]
              tunnel: w1979 -> [w2094]
              tunnel: [w2084] -> w1946 mode=indexing
              tunnel: [w2082] -> w1944 mode=indexing
              tunnel: [w2083] -> w1939 mode=indexing
              tunnel: w1965 -> [_]
              tunnel: [w2076] -> w1941 mode=indexing
              tunnel: [w2072] -> w1917 mode=indexing
              tunnel: [w2068] -> w1892 mode=indexing
              tunnel: [w2064] -> w1873 mode=indexing
              tunnel: [w2059] -> w1831 mode=indexing
              (unwired) TRUE ("line mode (F)")
              n1808 = Read from Text File "Read File"(file (use dialog)=w2095, error in=w2094) -> (text=w2060:string)  [unwired: 2 in, 3 out]
              n1809 = local write "String 7"(w2060) -> ()
              n1810 = String Subset(string=w2060, offset (0)=85, length (rest)=9 ("length (rest)")) -> (substring=w2063:string)
